vi "PD_Regulering.vi"(8 "k_d":dbl, 9 "k_p":dbl, 10 "SP":dbl, 11 "DATA":dbl) -> (0 "d_pd":dbl, 1 "p_pd":dbl, 2 "e(t)":dbl, 3 "u_pd":dbl)   [LabVIEW 2022 SP3]
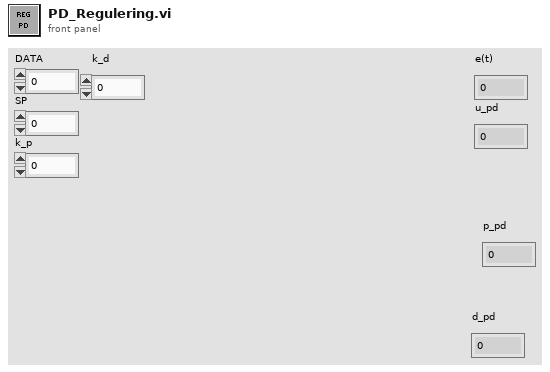
[diagram p1: front panel]
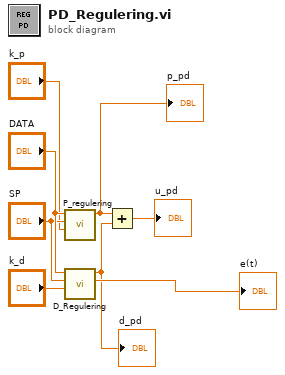
[diagram p0: block diagram]
diagram:
  n1 = call "P_regulering.vi"("k_p"="k_p", "SP"="SP", "DATA"="DATA") -> ("u_p"=w1:dbl)  [unwired: 6 in, 2 out]
  "p_pd" <- w1
  n2 = call "D_Regulering.vi"("k_d"="k_d", "SP"="SP", "DATA"="DATA") -> ("e(t)"=→"e(t)":dbl, "u_d"=w2:dbl)  [unwired: 7 in]
  "d_pd" <- w2
  n3 = Add(x=w1, y=w2) -> (x+y=→"u_pd":dbl)
